vi "Save to TDMS.vi"(8 "Error In":errorcluster, 10 "TDMS Ref":refnum<k34>, 11 "LHW-Data in":refnum<class "LHW-Data.lvclass">) -> (0 "Error Out":errorcluster, 3 "LHW-Data out":refnum<class "LHW-Data.lvclass">)   [LabVIEW 2014, in "LHW-Data.lvlib" / "LHW-Data.lvclass"]
doc: "Save data to TDMS file."
uses:
  LHW-Data.lvclass
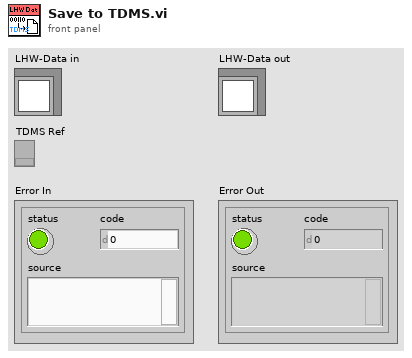
[diagram p1: front panel]
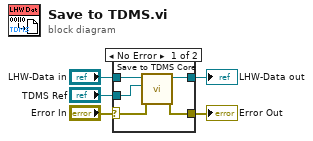
[diagram p0: block diagram]
diagram:
  n1 = case shown="No Error" "Error In" {
    selector: "Error In" -> [w7 w12]
    tunnel: [w6 w12] -> w4
    tunnel: [w9 w11] -> w2
    tunnel: "LHW-Data in" -> [w10 w11]
    tunnel: "TDMS Ref" -> [w8 _]
    frame No Error {
      n2 = call-dynamic "Save to TDMS Core.vi"("Error In"=w7, "TDMS Ref"=w8, "LHW-Data in"=w10) -> ("Error Out"=w6:errorcluster, "LHW-Data out"=w9:refnum<class "LHW-Data.lvclass">)  [unwired: 7 in]
    }
    frame Error {
    }
  }
  "Error Out" <- w4
  "LHW-Data out" <- w2
